vi "Switch Execute Test.vi"(6 "Driver Refs":T1, 7 "Colors":cluster{"Pass":u32, "Fail":u32, "Nop":u32}={"Pass"=6618880, "Fail"=16711680, "Nop"=16777226}, 8 "error in (no error)":errorcluster, 9 "Test Parameters In":T4) -> (0 "error out":errorcluster, 1 "Test Parameters Out":T4, 2 "Passed?":bool, 4 "dup Driver Ref":T1)   [LabVIEW 2011]
uses:
  TypeDefs/Switch Test Parameters.ctl
  TypeDefs/Switch Stimulus Parameters.ctl
  TypeDefs/Switch Type.ctl
  TypeDefs/Switch Instrument Info.ctl
  TypeDefs/Switch Driver Refs.ctl
  drivers/SWI/SWI Driver Ref.ctl
  drivers/PFE/PFE Driver Ref.ctl
  drivers/SWI/SWI Command.ctl
  drivers/PFE/PFE Command.ctl
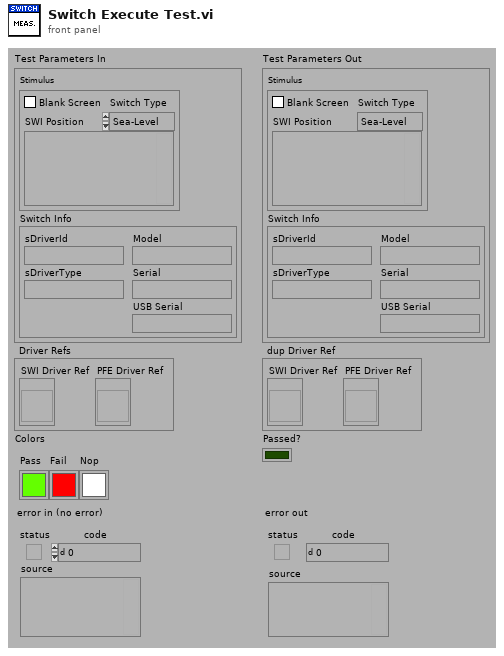
[diagram p1: front panel]
types:
  T1 = typedef "Switch Driver Refs.ctl" = cluster{"SWI Driver Ref":T2, "PFE Driver Ref":T3}
  T2 = typedef "SWI Driver Ref.ctl" = refnum<vi>
  T3 = typedef "PFE Driver Ref.ctl" = refnum<vi>
  T4 = typedef "Switch Test Parameters.ctl" = cluster{"Stimulus":T5, "Switch Info":T7}
  T5 = typedef "Switch Stimulus Parameters.ctl" = cluster{"Blank Screen":bool, "SWI Position":variant, "Switch Type":T6}
  T6 = typedef "Switch Type.ctl" = enum16{"Sea-Level", "Simulator", "SI-0206-SW", "SI-0309-SW", "SI-0310-SW", "Front End"}
  T7 = typedef "Switch Instrument Info.ctl" = cluster{"sDriverId":string, "sDriverType":string, "Model":string, "Serial":string, "USB Serial":string}
  T8 = typedef "SWI Command.ctl" = enum16{"LOAD", "INITIALIZE", "PRESET", "SET STIMULUS", "GET STIMULUS", "GET INFO", "RELEASE", "UNLOAD"}
  T9 = typedef "PFE Command.ctl" = enum16{"LOAD", "INITIALIZE", "PRESET", "SET STIMULUS", "GET STIMULUS", "GET INFO", "RELEASE", "UNLOAD"}
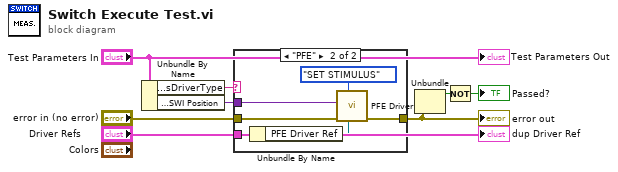
[diagram p0: block diagram]
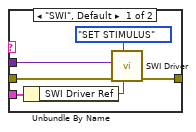
[diagram p2: hidden frame]
diagram:
  n1 = Unbundle By Name("Test Parameters In") -> ("Switch Info.sDriverType"=w2:string, "Stimulus.SWI Position"=w3:variant)
  n2 = case shown="\"PFE\"" w2 {
    tunnel: "error in (no error)" -> [w14 w20]
    tunnel: "Driver Refs" -> [w10 w16]
    tunnel: [w12 w18] -> w7
    tunnel: w3 -> [w11 w17]
    frame "SWI", Default {
      n3 = Unbundle By Name(w10) -> ("SWI Driver Ref"=w9:T2)
      n4 = call "SWI Driver.vi"("Drv Refnum"=w9, "SWI Command"=SWI_Command."SET STIMULUS", "error in (no error)"=w14, "SWI Position In"=w11) -> ("error out"=w12:errorcluster)  [unwired: 1 in, 6 out]
    }
    frame "PFE" {
      n5 = Unbundle By Name(w16) -> ("PFE Driver Ref"=w15:T3)
      n6 = call "PFE Driver.vi"("Drv Refnum"=w15, "PFE Command"=PFE_Command."SET STIMULUS", "error in (no error)"=w20, "PFE Position In"=w17) -> ("error out"=w18:errorcluster)  [unwired: 4 in, 3 out]
    }
  }
  "error out" <- w7
  n7 = Unbundle(w7) -> ("status"=w6:bool)  [unwired: 2 out]
  n8 = Not(x=w6) -> (.not. x?=→"Passed?":bool)
  "Test Parameters Out" <- "Test Parameters In"
  "dup Driver Ref" <- "Driver Refs"
